vi "auto_broadside_attack.vi"() -> ()   [LabVIEW 2012, in "2013-14.lvrbt"]
uses:
  2013-14.lvrbt
  <vilib>/NXT/Hardware/Plugins/Tetrix DC Motor/TetrixDCMotorAddress.ctl
  Drivers/AutoControlDirectAttack.ctl
  Drivers/AutoDriverControl.ctl
  <vilib>/NXT/HiTechnic/HiTechnic Controls/HiTechnic Port.ctl
  <vilib>/NXT/Block Support/NXT_InputPort.ctl
  FTC 2012 - 2013/Controls/SpeedControl.ctl
  <vilib>/NXT/NXTIO Xnodes/NXTIONodeSubVIs/TETRIX IO Check Battery.vi
  <vilib>/NXT/Dual Mode Library/Waits/Wait_Num(msec).vi
  <vilib>/NXT/NXTIO Xnodes/NXTIONodeSubVIs/TETRIX IO Stop DC Motors.vi
  <vilib>/NXT/Dual Mode Library/Display/drawText.vi
  <vilib>/NXT/Dual Mode Library/Sound/Tone.vi
  <vilib>/NXT/Subs/LVHSConnector.ctl
  <vilib>/NXT/NXTIO Xnodes/AddressXNode/NXTIOAddress.xnode
  AutoDirectAttack.lvrbt
  <vilib>/NXT/NXTIO Xnodes/NXTIOXNode/NXTIO.xnode
  <vilib>/NXT/LegoClasses/BrickReference/BrickReference.lvclass
panel:
  out "Enabled":bool
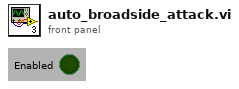
[diagram p1: front panel]
types:
  T1 = typedef "LVHSConnector.ctl" = refnum<class "BrickReference.lvclass">
  T2 = typedef "TetrixDCMotorAddress.ctl" = i16
  T3 = typedef "HiTechnic Port.ctl" = cluster{"Port":T4, "MUX Port":u8}
  T4 = typedef "NXT_InputPort.ctl" = u8
  T5 = typedef "AutoDriverControl.ctl" = enum16{"Init", "Forward", "Reverse", "Left", "Right", "Brake"}
  T6 = typedef "AutoControlDirectAttack.ctl" = enum16{"FindIRBasket", "ApproachLeft", "ApproachRight", "AlignCrate", "DropBLK", "DrvToEndOfBaskets", "DrvAroundBaskets", "AlignWithRamp", "ParkOnRamp"}
  T7 = cluster{"TetrixDCMotor":T2, "TetrixDCMotor 2":T2}
  T8 = typedef "SpeedControl.ctl" = enum16{"Fast", "Medium", "Slow"}
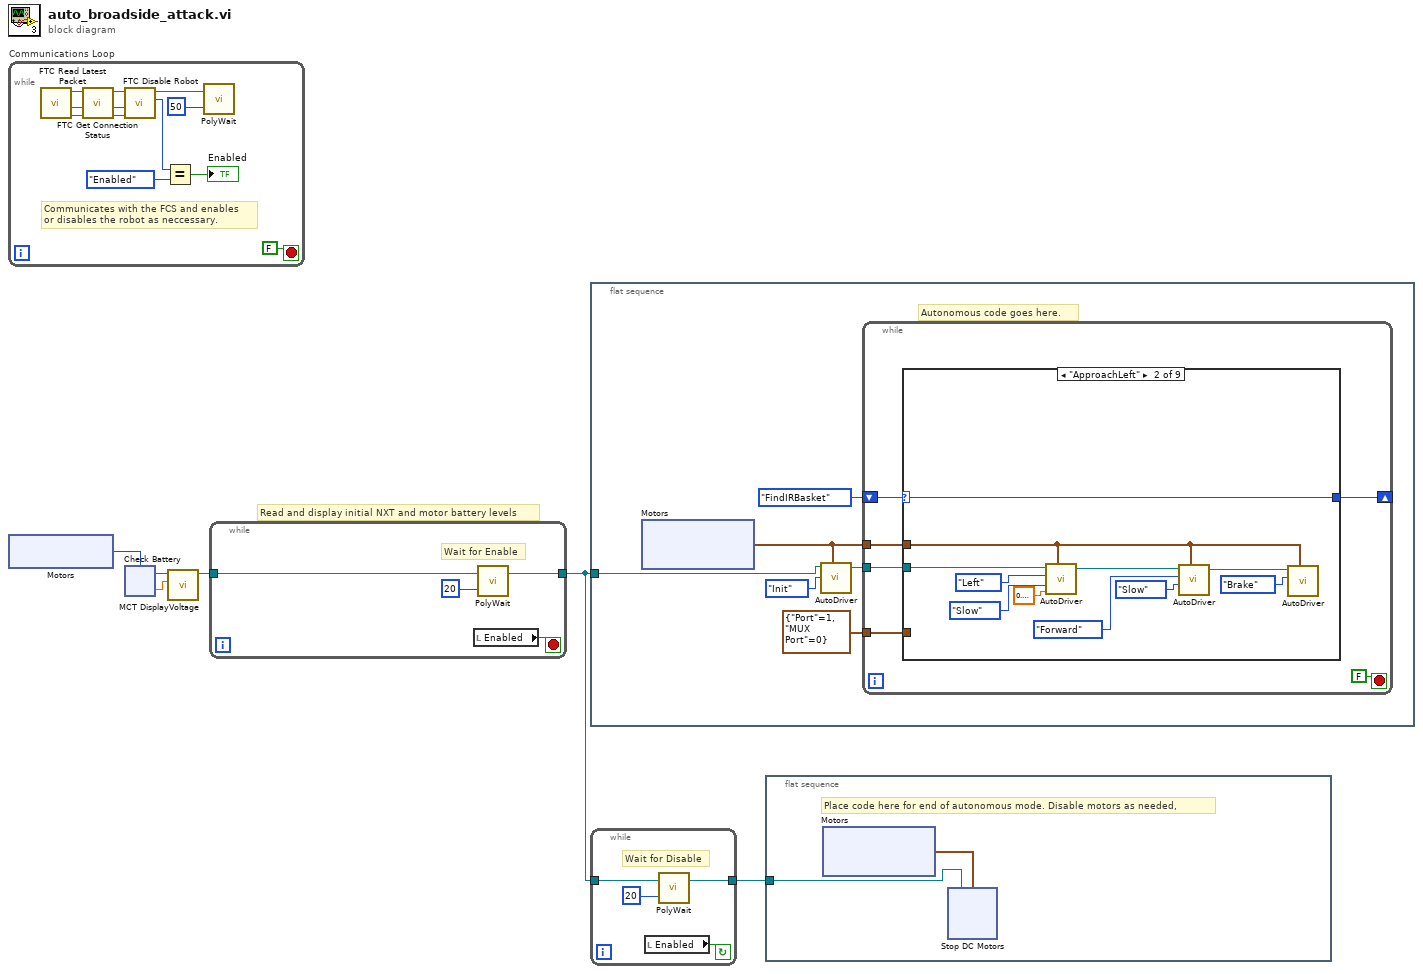
[diagram p0: block diagram]
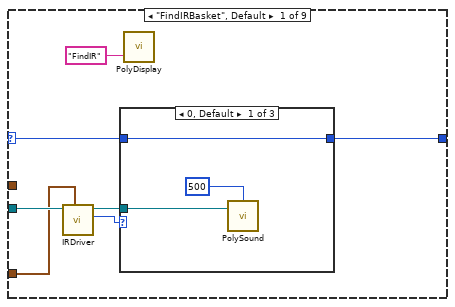
[diagram p2: hidden frame]
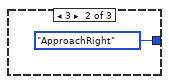
[diagram p3: hidden frame]
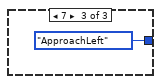
[diagram p4: hidden frame]
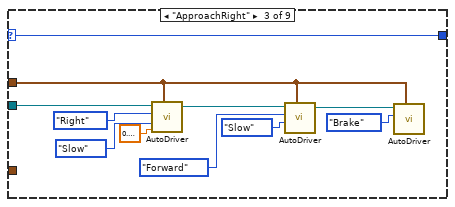
[diagram p5: hidden frame]
diagram:
  # "Read and display initial NXT and motor battery levels"
  n1 = while "Communications Loop" {
    stop <- FALSE stop-if-true
    # "Communicates with the FCS and enables \nor disables the robot as neccessary."
    n2 = call <vilib>:"FTC Read Latest Packet.vi"() -> ("Packet Received?"=w16:bool, "Stopped?"=w15:bool, "NXT"=w18:T1)  [unwired: 6 in, 3 out]
    n3 = call <vilib>:"FTC Get Connection Status.vi"("Packet Received?"=w16, "Stopped?"=w15, "NXT"=w18) -> ("Online?"=w7:bool, "Stopped?"=w8:bool, "NXT"=w17:T1)  [unwired: 5 in]
    n4 = call <vilib>:"FTC Disable Robot.vi"("Online?"=w7, "Stopped?"=w8, "NXT"=w17) -> ("Enabled?"=w11:enum16{"Disabled", "Enabled"}, "NXT"=w13:T1)  [unwired: 3 in]
    n5 = Equal?(x=w11, y=enum16{"Disabled", "Enabled"}."Enabled") -> (x = y?=→"Enabled":bool)
    n6 = call-poly <vilib>:"PolyWait.vi"("Time (100 msec)"=u32 50 ("Time (msec)"), "NXT"=w13) -> ()  [unwired: 2 in, 1 out]
  }
  n7 = xnode "Motors"() -> ("Motor"=w6:T2)
  n8 = xnode "Check Battery"("Motors"=w6) -> ("Voltage 1"=w1:sgl, "NXT"=w3:T1)  [unwired: 1 in]
  n9 = call <vilib>:"MCT DisplayVoltage.vi"("Motor Voltage"=w1, "NXT"=w3) -> ("NXT"=w2:T1)  [unwired: 9 in]
  n10 = while {
    tunnel: [w20] -> w5
    tunnel: w2 -> [w19]
    stop <- w21 stop-if-true
    # "Wait for Enable"
    n11 = local read "Enabled"() -> (w21:bool)
    n12 = call-poly <vilib>:"PolyWait.vi"("Time (100 msec)"=u32 20 ("Time (msec)"), "NXT"=w19) -> ("NXT"=w20:T1)  [unwired: 2 in]
  }
  n13 = flat-sequence {
    tunnel: w5 -> [w27]
    frame #0 {
      # "Autonomous code goes here."
      n14 = xnode "Motors"() -> ("Motor"=w23:cluster{"TetrixDCMotor":T2, "TetrixDCMotor":T2})
      n15 = call "AutoDriver.vi"("NXT In"=w27, "Motors"=w23, "Direction"=AutoDriverControl."Init") -> ("NXT Out"=w25:T1)  [unwired: 5 in]
      n16 = while {
        shift-right: [w32] -> _
        shift-left: AutoControlDirectAttack."FindIRBasket" ("AutoControl") -> [w34]
        tunnel: w25 -> [w33]
        tunnel: T3 {"Port"=1, "MUX Port"=0} ("Port") -> [w31]
        tunnel: w23 -> [w30]
        stop <- FALSE stop-if-true
        n17 = case shown="\"ApproachLeft\"" w34 {
          selector: w34 -> [w38 w58 w69 w70 w71 w72 w73 w74 w75]
          tunnel: w33 -> [w42 w49 w60 _ _ _ _ _ _]
          tunnel: [w37 w58 w69 w70 w71 w72 w73 w74 w75] -> w32
          tunnel: w31 -> [w41 _ _ _ _ _ _ _ _]
          tunnel: w30 -> [_ w48 w59 _ _ _ _ _ _]
          frame "FindIRBasket", Default {
            n18 = call "IRDriver.vi"("Port"=w41, "NXT In"=w42) -> ("Sector (0-9)"=w40:i16, "NXT Out"=w39:T1)  [unwired: 8 in]
            n19 = case shown="0, Default" w40 {
              tunnel: w39 -> [w44 _ _]
              tunnel: w38 -> [w43 _ _]
              tunnel: [w43 AutoControlDirectAttack."ApproachRight" ("AutoControl") AutoControlDirectAttack."ApproachLeft" ("AutoControl")] -> w37
              frame 0, Default {
                n20 = call-poly <vilib>:"PolySound.vi"("NXT"=w44, "Tone (440 Hz)"=u16 500) -> ()  [unwired: 2 in, 1 out]
              }
              frame 3 {
              }
              frame 7 {
              }
            }
            n21 = call-poly <vilib>:"PolyDisplay.vi"("Text"="FindIR") -> ()  [unwired: 3 in, 1 out]
          }
          frame "ApproachLeft" {
            n22 = call "AutoDriver.vi"("NXT In"=w49, "Motors"=w48, "Direction"=AutoDriverControl."Left", "Speed"=SpeedControl."Slow", "Time (1 sec)"=sgl 0.3) -> ("NXT Out"=w54:T1)  [unwired: 3 in]
            n23 = call "AutoDriver.vi"("NXT In"=w54, "Motors"=w48, "Direction"=AutoDriverControl."Forward", "Speed"=SpeedControl."Slow") -> ("NXT Out"=w51:T1)  [unwired: 4 in]
            n24 = call "AutoDriver.vi"("NXT In"=w51, "Motors"=w48, "Direction"=AutoDriverControl."Brake") -> ()  [unwired: 5 in, 1 out]
          }
          frame "ApproachRight" {
            n25 = call "AutoDriver.vi"("NXT In"=w60, "Motors"=w59, "Direction"=AutoDriverControl."Right", "Speed"=SpeedControl."Slow", "Time (1 sec)"=sgl 0.3) -> ("NXT Out"=w65:T1)  [unwired: 3 in]
            n26 = call "AutoDriver.vi"("NXT In"=w65, "Motors"=w59, "Direction"=AutoDriverControl."Forward", "Speed"=SpeedControl."Slow") -> ("NXT Out"=w62:T1)  [unwired: 4 in]
            n27 = call "AutoDriver.vi"("NXT In"=w62, "Motors"=w59, "Direction"=AutoDriverControl."Brake") -> ()  [unwired: 5 in, 1 out]
          }
          frame "AlignCrate" {
          }
          frame "DropBLK" {
          }
          frame "DrvToEndOfBaskets" {
          }
          frame "DrvAroundBaskets" {
          }
          frame "AlignWithRamp" {
          }
          frame "ParkOnRamp" {
          }
        }
      }
    }
  }
  n28 = while {
    tunnel: [w77] -> w4
    tunnel: w5 -> [w76]
    stop <- w78 continue-if-true
    # "Wait for Disable"
    n29 = local read "Enabled"() -> (w78:bool)
    n30 = call-poly <vilib>:"PolyWait.vi"("Time (100 msec)"=u32 20 ("Time (msec)"), "NXT"=w76) -> ("NXT"=w77:T1)  [unwired: 2 in]
  }
  n31 = flat-sequence {
    tunnel: w4 -> [w81]
    frame #0 {
      # "Place code here for end of autonomous mode. Disable motors as needed,"
      n32 = xnode "Motors"() -> ("Motor"=w80:cluster{"TetrixDCMotor":T2, "TetrixDCMotor":T2})
      n33 = xnode "Stop DC Motors"("Motors"=w80, "NXT"=w81) -> ()  [unwired: 1 out]
    }
  }
